vi "Get IO Level.vi"(8 "error in (no error)":errorcluster, 10 "iLevel":i32, 11 "index":i32) -> (0 "error out":errorcluster, 2 "iLevel out":i32, 3 "function return":u32)   [LabVIEW 2014, in "atmcd32d.lvlib"]
doc: "unsigned int WINAPI GetIOLevel(int index, int * iLevel);"
uses:
  atmcd32d.lvlib
  atmcd32d.dll
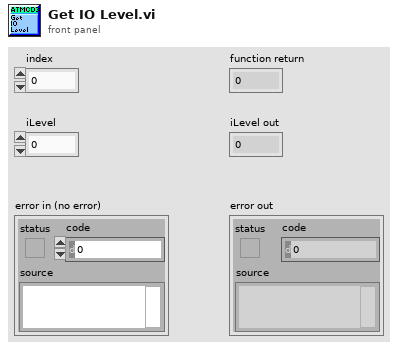
[diagram p1: front panel]
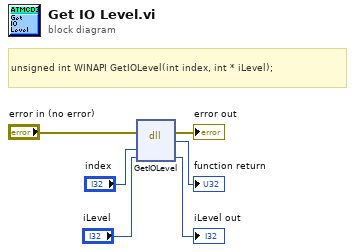
[diagram p0: block diagram]
diagram:
  # "unsigned int WINAPI GetIOLevel(int index, int * iLevel);"
  n1 = dll-call lib="C:/Users/Bakir/Documents/Lambda2-Testing/lib/Andorlib/atmcd32d.*" fn="GetIOLevel"(error in="error in (no error)", "index"="index", "iLevel"="iLevel") -> (error out=→"error out":errorcluster, →"function return":u32, "iLevel"=→"iLevel out":i32)  [unwired: 3 in, 1 out]
